vi "PART_II_main.vi"() -> ()   [LabVIEW 2019]
uses:
  <vilib>/sound2/lvsound2.llb/Sampling Mode.ctl
  <vilib>/sound2/lvsound2.llb/Sound Data Format.ctl
  <vilib>/sound2/lvsound2.llb/Sound Input Read (DBL).vi
panel:
  out "x > y":bool
  out "Current Data around Peak":dbl[](graph)
  out "max index(es)":i32
  out "Multiple Found Data":dbl[][](graph)
  out "Mean and Confidence Intervals":dbl[][](graph)
  in  "Window Length":i32=200
  out "Max Just Found":bool
  in  "Threshold":dbl=0.005
  out "Raw Data":waveform(dbl)[](graph)
  in  "Stop":bool
  in  "Device ID":u32 format="%.0x"
  in  "Number of Samples/ch":i32=2000
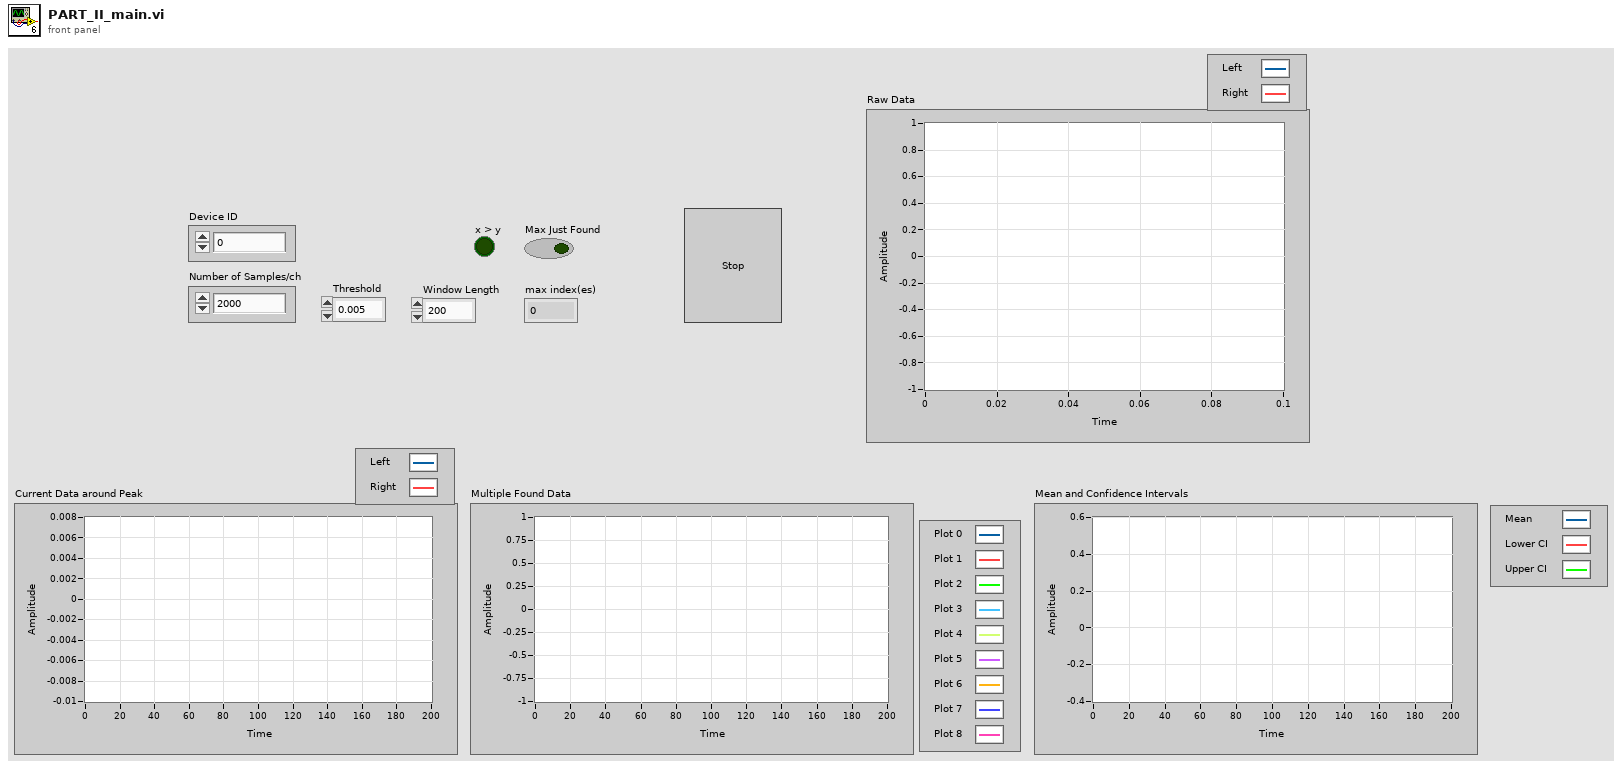
[diagram p1: front panel]
types:
  T1 = typedef "Sound Data Format.ctl" = cluster{"sample rate (S/s)":dbl, "number of channels":i32, "bits per sample":i32}
  T2 = typedef "Sampling Mode.ctl" = i32
  T3 = typedef "Sound Input Task ID.ctl" = u32
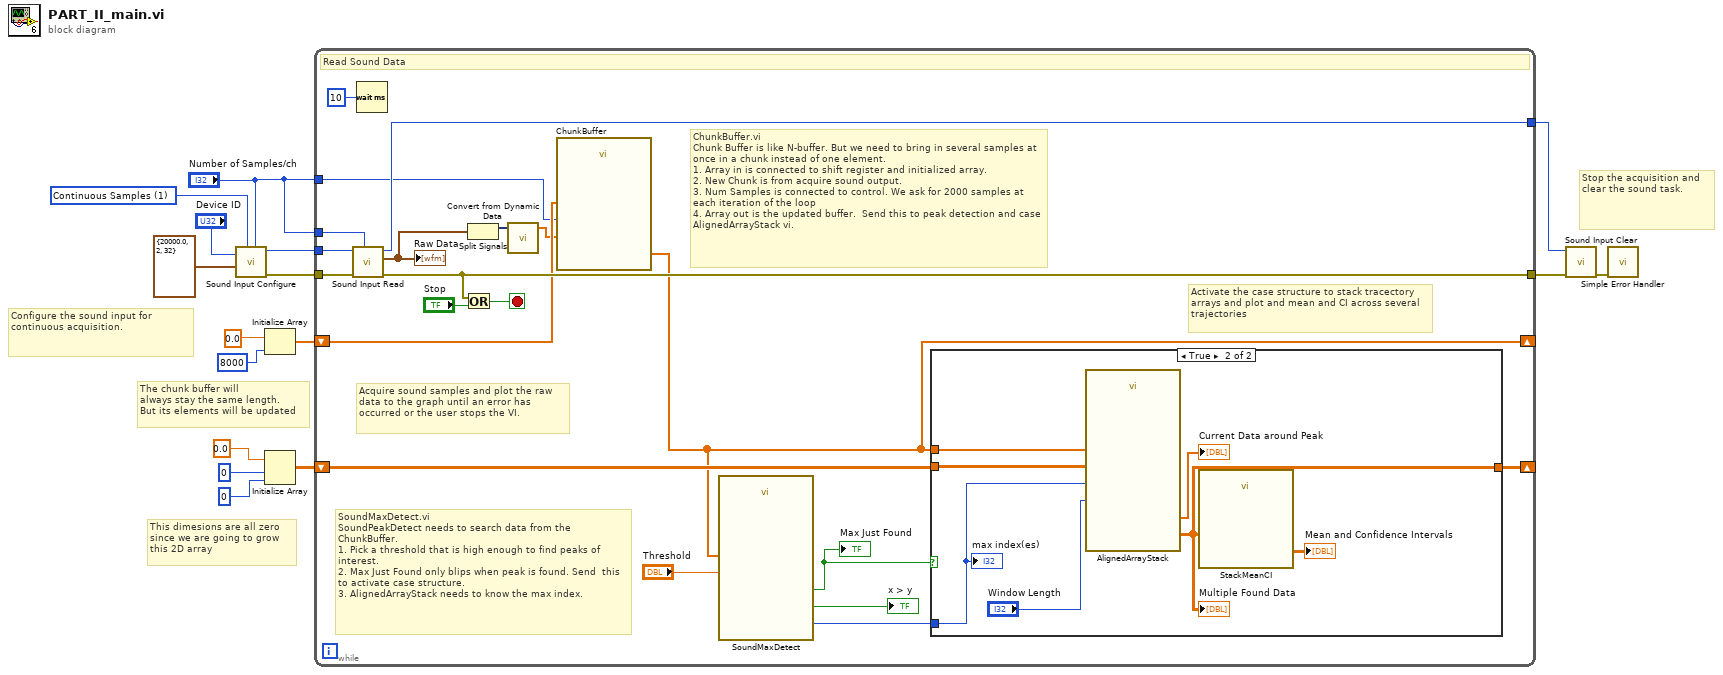
[diagram p0: block diagram]
diagram:
  w11 = T2 1 items=["Finite Samples", "Continuous Samples"] ("sample mode")
  # "The chunk buffer will\nalways stay the same length.\nBut its elements will be updated"
  # "This dimesions are all zero\nsince we are going to grow \nthis 2D array"
  # "Stop the acquisition and clear the sound task."
  # "Configure the sound input for continuous acquisition."
  n1 = call <vilib>:"Sound Input Configure.vi"("number of samples/ch"="Number of Samples/ch", "sample mode"=w11, "sound format"=T1 {"sample rate (S/s)"=20000.0, "number of channels"=2, "bits per sample"=32} ("Sound Format"), "device ID"="Device ID") -> ("error out"=w16:errorcluster, "task ID"=w14:T3)  [unwired: 6 in]
  n2 = Initialize Array(0.0 ("element"), 8000 ("dimension size")) -> (w3:dbl[])
  n3 = Initialize Array(0.0 ("element"), 0 ("dimension size"), 0 ("dimension size")) -> (w1:dbl[][])
  n4 = while {
    tunnel: w14 -> [w35]
    tunnel: [w34] -> w13
    tunnel: "Number of Samples/ch" -> [w33]
    tunnel: w16 -> [w36]
    tunnel: [w30] -> w12
    shift-right: [w17] -> _
    shift-left: w3 -> [w25]
    tunnel: "Number of Samples/ch" -> [w24]
    shift-right: [w18] -> _
    shift-left: w1 -> [w20]
    stop <- w31 stop-if-true
    # "Activate the case structure to stack tracectory arrays and plot and mean and CI across several trajectories"
    # "SoundMaxDetect.vi\nSoundPeakDetect needs to search data from the ChunkBuffer. \n1. Pick a threshold that is high enough to find peaks of interest.\n2. Max Just Found only blips when peak is found. Send  this to activate case structure.\n3. AlignedArrayStack needs to know the max index."
    # "ChunkBuffer.vi\nChunk Buffer is like N-buffer. But we need to bring in several samples at once in a chunk instead of one element. \n1. Array in is connected to shift register and initialized array.\n2. New Chunk is from acquire sound output.\n3. Num Samples is connected to control. We ask for 2000 samples at each iteration of the loop\n4. Array out is the updated buffer.  Send this to peak detection and case AlignedArrayStack vi."
    # "Acquire sound samples and plot the raw data to the graph until an error has occurred or the user stops the VI."
    # "Read Sound Data"
    n5 = call-poly <vilib>:"Sound Input Read.vi"("number of samples/ch"=w33, "error in (no error)"=w36, "task ID"=w35) -> ("error out"=w30:errorcluster, "data"=w29:waveform(dbl)[], "task ID out"=w34:T3)  [unwired: 6 in]
    "Raw Data" <- w29
    n6 = Wait (ms)(milliseconds to wait=u32 10) -> ()  [unwired: 1 out]
    n7 = Or(x=w30, y="Stop") -> (x .or. y?=w31:bool)
    n8 = Split Signals(w29) -> (w28:dynamicdata)  [unwired: 2 in, 1 out]
    n9 = call "Convert from Dynamic Data"("Dynamic Data Type"=w28) -> ("Array"=w23:dbl[])  [unwired: 3 in]
    n10 = call "ChunkBuffer.vi"("Array in"=w25, "Chunk Length"=w24, "New Chunk in"=w23) -> ("Array out"=w17:dbl[])  [unwired: 8 in]
    n11 = call "SoundMaxDetect.vi"("Threshold"="Threshold", "Buffer In"=w17) -> ("Just Changed"=w21:bool, "Max Found"=→"x > y":bool, "Peak Index"=w19:i32)  [unwired: 7 in]
    "Max Just Found" <- w21
    n12 = case shown="True" w21 {
      tunnel: w20 -> [w37 w41]
      tunnel: w17 -> [_ w40]
      tunnel: w19 -> [_ w38]
      tunnel: [w37 w39] -> w18
      frame False {
      }
      frame True {
        n13 = call "AlignedArrayStack.vi"("Window Length"="Window Length", "Peak Index"=w38, "Old Stack"=w41, "New Trace"=w40) -> ("New Stack"=w39:dbl[][], "Mini Window"=→"Current Data around Peak":dbl[])  [unwired: 6 in]
        "Multiple Found Data" <- w39
        n14 = call "StackMeanCI.vi"("Stack"=w39) -> ("Three Lines"=→"Mean and Confidence Intervals":dbl[][])  [unwired: 10 in]
        "max index(es)" <- w38
      }
    }
  }
  n15 = call <vilib>:"Sound Input Clear.vi"("error in (no error)"=w12, "task ID"=w13) -> ("error out"=w10:errorcluster)  [unwired: 9 in]
  n16 = call <vilib>:"Simple Error Handler.vi"("error in (no error)"=w10) -> ()  [unwired: 4 in, 5 out]
